vi "Host.vi"() -> ()   [LabVIEW 2018]
uses:
  <instrlib>/niDCPower/nidcpower.llb/niDCPower Measurement Type.ctl
panel:
  in  "Ток, LED":dbl=0.1 caption="current limit" format="%.6p"
  in  "Свет":bool caption="output enabled"
  in  "LED, V":dbl=6.0 caption="voltage level" format="%_6p"
  in  "Период опроса, мс":u32=1
  in  "1.1, V":dbl=7.0 caption="voltage level" format="%_6p"
  in  "Ток, A":dbl=1.0 caption="current limit" format="%_6p"
  in  "Стоп":bool
  in  "Питание":bool
  in  "SEL_T, мс":u32=100
  in  "SIM_SEL":bool
  out "SEL":bool
  in  "27_selcur":dbl=0.3 caption="current limit" format="%_6p"
  out "27":i32
  out "27":bool
  out "27_cur, A":dbl caption="measurement" format="%_6g"
  in  "0.1, V":dbl=20.0 caption="voltage level" format="%_6p"
  out "27 Chart":dbl(graph)=0.0024647493843340824
  in  "0.1":refnum<k15>="PXI1Slot2" caption="instrument handle"
  in  "1.1":refnum<k15>="PXI1Slot3" caption="instrument handle"
  in  "SEL":path=path "C:/LabView_PRJ/24138_Electron/SEL"
  out "Номер образца":string="0"
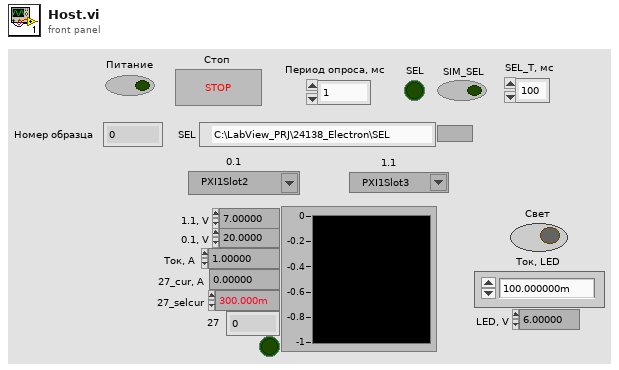
[diagram p1: front panel]
types:
  T1 = enum16{"open", "replace", "create", "open or create", "replace or create", "replace or create with confirmation"}
  T2 = typedef "niDCPower Measurement Type.ctl" = i32
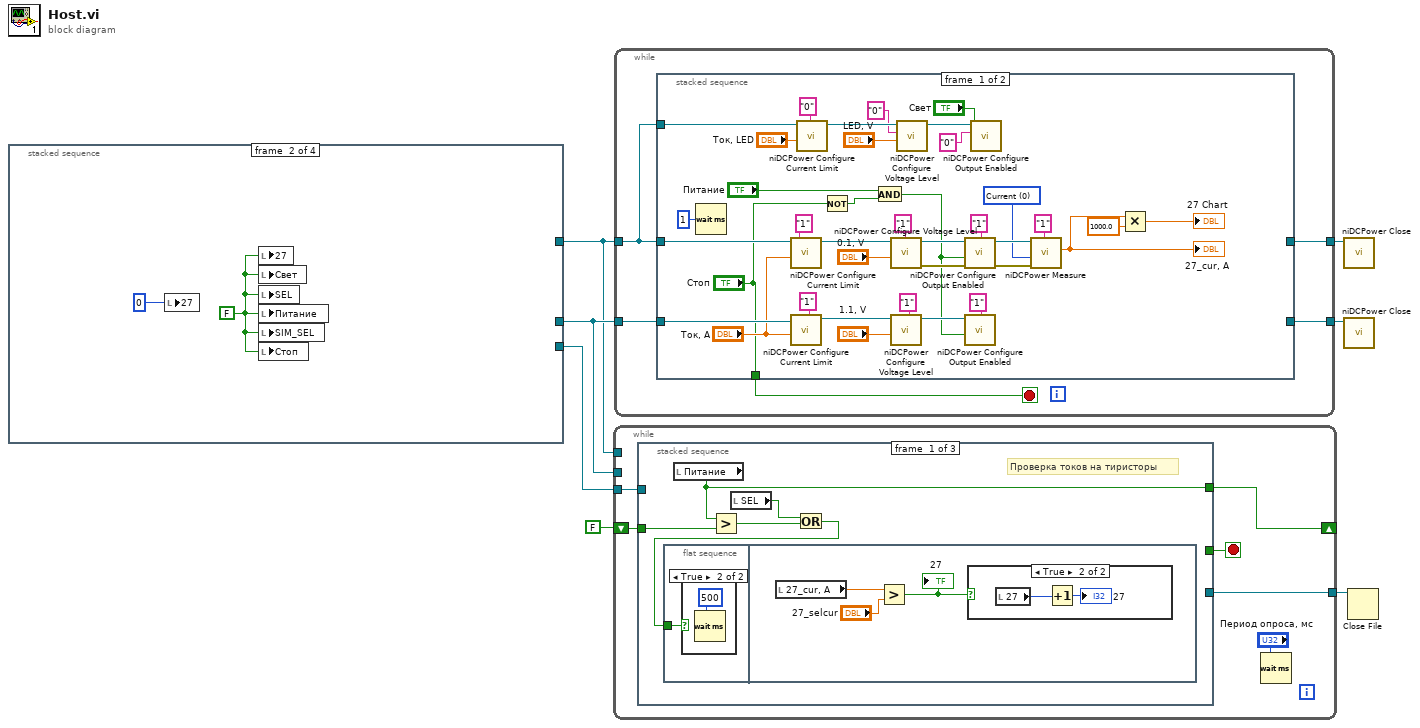
[diagram p0: block diagram]
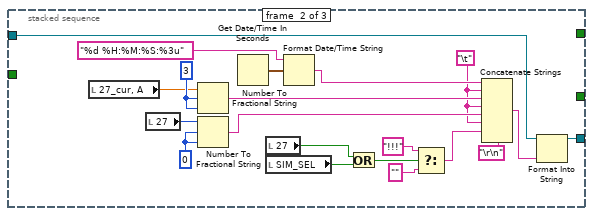
[diagram p4: hidden frame]
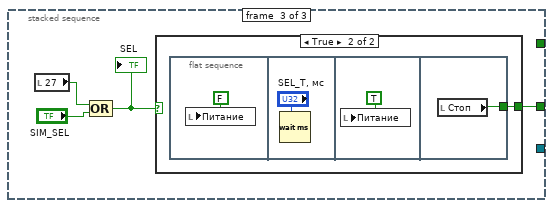
[diagram p5: hidden frame]
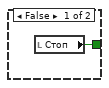
[diagram p6: hidden frame]
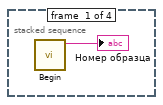
[diagram p8: hidden frame]
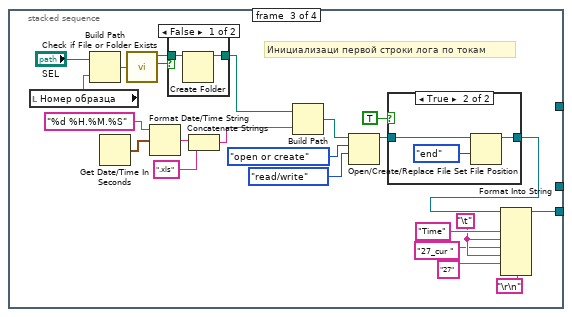
[diagram p9: hidden frame]
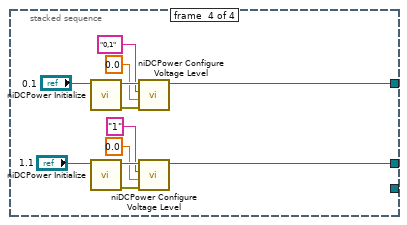
[diagram p12: hidden frame]
diagram:
  n1 = stacked-sequence {
    tunnel: [_ _ _ w42] -> w4
    tunnel: [_ _ _ w41] -> w3
    tunnel: [_ _ w17 _] -> w6
    frame #0 {
      n2 = call "Begin.vi"() -> ("Номер образца 2"=→"Номер образца":string)  [unwired: 11 in]
    }
    frame #1 {
      w10 = FALSE
      n3 = local write "27"(0) -> ()
      n4 = local write "27"(w10) -> ()
      n5 = local write "Свет"(w10) -> ()
      n6 = local write "SEL"(w10) -> ()
      n7 = local write "Питание"(w10) -> ()
      n8 = local write "SIM_SEL"(w10) -> ()
      n9 = local write "Стоп"(w10) -> ()
    }
    frame #2 {
      w14 = "\t"
      # "Инициализаци первой строки лога по токам"
      n10 = local read "Номер образца"() -> (w29:string)
      n11 = Build Path(base path="SEL", name or relative path=w29) -> (appended path=w31:path)
      n12 = Get Date/Time In Seconds() -> (seconds since 1Jan1904=w24:timestamp)
      n13 = call <vilib>:"Check if File or Folder Exists.vi"("path"=w31) -> ("file or folder exists?"=w32:bool, "dup path"=w33:path)  [unwired: 8 in, 1 out]
      n14 = Format Date/Time String(time format string (%c)="%d %H.%M.%S", seconds (now)=w24) -> (date/time string=w21:string)  [unwired: 1 in]
      n15 = case shown="False" w32 {
        tunnel: w33 -> [w39 w40]
        tunnel: [w38 w40] -> w16
        frame False {
          n16 = Create Folder(path (use dialog)=w39) -> (created path=w38:path)  [unwired: 2 in, 2 out]
        }
        frame True {
        }
      }
      n17 = Concatenate Strings(w21, ".xls" ("string")) -> (w19:string)
      n18 = Build Path(base path=w16, name or relative path=w19) -> (appended path=w22:path)
      n19 = Open/Create/Replace File(file path (use dialog)=w22, operation (0:open)=T1."open or create", access (0:read/write)=enum16{"read/write", "read-only", "write-only"}."read/write") -> (refnum out=w25:refnum<file>)  [unwired: 3 in, 2 out]
      n20 = case shown="True" TRUE {
        tunnel: w25 -> [w34 w37]
        tunnel: [w34 w35] -> w18
        frame False {
        }
        frame True {
          n21 = Set File Position(refnum=w37, from (0:start)=enum16{"start", "end", "current"}."end") -> (refnum out=w35:refnum<file>)  [unwired: 2 in, 1 out]
        }
      }
      n22 = Format Into String(initial string=w18, "Time" ("input 1"), w14, "27_cur " ("input 1"), w14, "27" ("input 1"), "\r\n") -> (resulting string=w17:refnum<file>)  [unwired: 2 in, 1 out]
    }
    frame #3 {
      n23 = call <instrlib>:"niDCPower Initialize.vi"("resource name"="0.1") -> ("error out"=w49:errorcluster, "instrument handle out"=w51:refnum<k15>)  [unwired: 3 in, 6 out]
      n24 = call <instrlib>:"niDCPower Initialize.vi"("resource name"="1.1") -> ("error out"=w50:errorcluster, "instrument handle out"=w52:refnum<k15>)  [unwired: 3 in, 6 out]
      n25 = call <instrlib>:"niDCPower Configure Voltage Level.vi"("error in (no error)"=w49, "voltage level"=0.0, "channel name"="0,1", "instrument handle"=w51) -> ("instrument handle out"=w41:refnum<k15>)  [unwired: 6 in, 1 out]
      n26 = call <instrlib>:"niDCPower Configure Voltage Level.vi"("error in (no error)"=w50, "voltage level"=0.0, "channel name"="1", "instrument handle"=w52) -> ("instrument handle out"=w42:refnum<k15>)  [unwired: 6 in, 1 out]
    }
  }
  n27 = while {
    shift-right: [w58] -> _
    shift-left: FALSE -> [w57]
    tunnel: w6 -> [w56]
    tunnel: [w54] -> w5
    tunnel: w4 -> [_]
    tunnel: w3 -> [_]
    stop <- w55 stop-if-true
    n28 = stacked-sequence {
      tunnel: [w62 _ _] -> w58
      tunnel: w57 -> [w63 _ _]
      tunnel: w56 -> [_ w85 _]
      tunnel: [_ _ w94] -> w55
      tunnel: [_ w84 _] -> w54
      frame #0 {
        # "Проверка токов на тиристоры"
        n29 = flat-sequence {
          tunnel: w59 -> [w64]
          frame #0 {
            n30 = case shown="True" w64 {
              frame False {
              }
              frame True {
                n31 = Wait (ms)(milliseconds to wait=u32 500) -> ()  [unwired: 1 out]
              }
            }
          }
          frame #1 {
            n32 = local read "27_cur, A"() -> (w66:dbl)
            n33 = Greater?(x=w66, y="27_selcur") -> (0:w67:bool)
            "27" <- w67
            n34 = case shown="True" w67 {
              frame False {
              }
              frame True {
                n35 = local read "27"() -> (w70:i32)
                n36 = Increment(x=w70) -> (x+1=→"27":i32)
              }
            }
          }
        }
        n37 = local read "Питание"() -> (w62:bool)
        n38 = Greater?(x=w62, y=w63) -> (0:w61:bool)
        n39 = local read "SEL"() -> (w60:bool)
        n40 = Or(x=w60, y=w61) -> (x .or. y?=w59:bool)
      }
      frame #1 {
        w82 = i16 0 ("width (-)")
        w83 = i16 3 ("width (-)")
        w73 = "\t"
        n41 = local read "27_cur, A"() -> (w75:dbl)
        n42 = local read "27"() -> (w81:i32)
        n43 = Number To Fractional String(number=w75, width (-)=w83, precision (6)=w83) -> (F-format string=w79:string)  [unwired: 1 in]
        n44 = Number To Fractional String(number=w81, width (-)=w82, precision (6)=w82) -> (F-format string=w74:string)  [unwired: 1 in]
        n45 = Get Date/Time In Seconds() -> (seconds since 1Jan1904=w90:timestamp)
        n46 = local read "27"() -> (w77:bool)
        n47 = local read "SIM_SEL"() -> (w76:bool)
        n48 = Format Date/Time String(time format string (%c)="%d %H:%M:%S:%3u", seconds (now)=w90) -> (date/time string=w80:string)  [unwired: 1 in]
        n49 = Or(x=w77, y=w76) -> (x .or. y?=w78:bool)
        n50 = Select(t="!!!", s=w78, f="") -> (s? t:f=w72:string)
        n51 = Concatenate Strings(w80, w73, w79, w73, w74, w73, w72, "\r\n") -> (w89:string)
        n52 = Format Into String(initial string=w85, w89) -> (resulting string=w84:refnum<file>)  [unwired: 2 in, 1 out]
      }
      frame #2 {
        n53 = local read "27"() -> (w92:bool)
        n54 = Compound Arithmetic op=OR(w92, "SIM_SEL") -> (w93:bool)
        "SEL" <- w93
        n55 = case shown="True" w93 {
          tunnel: [w95 w96] -> w94
          frame False {
            n56 = local read "Стоп"() -> (w95:bool)
          }
          frame True {
            n57 = flat-sequence {
              tunnel: [w100] -> w96
              frame #0 {
                n58 = local write "Питание"(FALSE ("SYS_RESET")) -> ()
              }
              frame #1 {
                n59 = Wait (ms)(milliseconds to wait="SEL_T, мс") -> ()  [unwired: 1 out]
              }
              frame #2 {
                n60 = local write "Питание"(TRUE ("SYS_RESET")) -> ()
              }
              frame #3 {
                n61 = local read "Стоп"() -> (w100:bool)
              }
            }
          }
        }
      }
    }
    n62 = Wait (ms)(milliseconds to wait="Период опроса, мс") -> ()  [unwired: 1 out]
  }
  n63 = while {
    tunnel: w3 -> [w101]
    tunnel: w4 -> [w105]
    tunnel: [w104] -> w2
    tunnel: [w103] -> w1
    stop <- w102 stop-if-true
    n64 = stacked-sequence {
      tunnel: w105 -> [w124 w143]
      tunnel: w101 -> [w123 w144]
      tunnel: [_ w144] -> w104
      tunnel: [_ w143] -> w103
      tunnel: ["Стоп" _] -> w102
      tunnel: w101 -> [w114 _]
      frame #0 {
        w125 = T2 0 items=["Current", "Voltage"] ("measurement type")
        n65 = Wait (ms)(milliseconds to wait=u32 1) -> ()  [unwired: 1 out]
        n66 = call <instrlib>:"niDCPower Configure Current Limit.vi"("current limit"="Ток, A", "channel name"="1", "instrument handle"=w123) -> ("instrument handle out"=w137:refnum<k15>)  [unwired: 7 in, 1 out]
        n67 = call <instrlib>:"niDCPower Configure Current Limit.vi"("current limit"="Ток, A", "channel name"="1", "instrument handle"=w124) -> ("instrument handle out"=w129:refnum<k15>)  [unwired: 7 in, 1 out]
        n68 = call <instrlib>:"niDCPower Configure Current Limit.vi"("current limit"="Ток, LED", "channel name"="0", "instrument handle"=w114) -> ("instrument handle out"=w113:refnum<k15>)  [unwired: 7 in, 1 out]
        n69 = Not(x="Стоп") -> (.not. x?=w117:bool)
        n70 = And(x="Питание", y=w117) -> (x .and. y?=w115:bool)
        n71 = call <instrlib>:"niDCPower Configure Voltage Level.vi"("voltage level"="0.1, V", "channel name"="1", "instrument handle"=w137) -> ("error out"=w135:errorcluster, "instrument handle out"=w136:refnum<k15>)  [unwired: 7 in]
        n72 = call <instrlib>:"niDCPower Configure Voltage Level.vi"("voltage level"="1.1, V", "channel name"="1", "instrument handle"=w129) -> ("instrument handle out"=w127:refnum<k15>)  [unwired: 7 in, 1 out]
        n73 = call <instrlib>:"niDCPower Configure Voltage Level.vi"("voltage level"="LED, V", "channel name"="0", "instrument handle"=w113) -> ("instrument handle out"=w112:refnum<k15>)  [unwired: 7 in, 1 out]
        n74 = call <instrlib>:"niDCPower Configure Output Enabled.vi"("error in (no error)"=w135, "output enabled"=w115, "channel name"="1", "instrument handle"=w136) -> ("error out"=w138:errorcluster, "instrument handle out"=w139:refnum<k15>)  [unwired: 6 in]
        n75 = call <instrlib>:"niDCPower Configure Output Enabled.vi"("output enabled"=w115, "channel name"="1", "instrument handle"=w127) -> ()  [unwired: 7 in, 2 out]
        n76 = call <instrlib>:"niDCPower Configure Output Enabled.vi"("output enabled"="Свет", "channel name"="0", "instrument handle"=w112) -> ()  [unwired: 7 in, 2 out]
        n77 = call <instrlib>:"niDCPower Measure.vi"("error in (no error)"=w138, "measurement type"=w125, "channel name"="1", "instrument handle"=w139) -> ("measurement"=w119:dbl)  [unwired: 5 in, 2 out]
        "27_cur, A" <- w119
        n78 = Multiply(x=w119, y=1000.0) -> (x*y=→"27 Chart":dbl)
      }
      frame #1 {
      }
    }
  }
  n79 = call <instrlib>:"niDCPower Close.vi"("instrument handle"=w2) -> ()  [unwired: 10 in, 1 out]
  n80 = call <instrlib>:"niDCPower Close.vi"("instrument handle"=w1) -> ()  [unwired: 10 in, 1 out]
  n81 = Close File(refnum=w5) -> ()  [unwired: 1 in, 2 out]
